vi "Main.vi"(8 "Error in":errorcluster) -> (0 "error out":errorcluster)   [LabVIEW 2018, in "Module B.lvlib"]
uses:
  Module B.lvlib
  Private/ctl/Message Data--cluster.ctl
  Private/ctl/State--enum.ctl
  Common/Common.lvlib
panel:
  out "Msg":string
  in  "Shut module A":bool
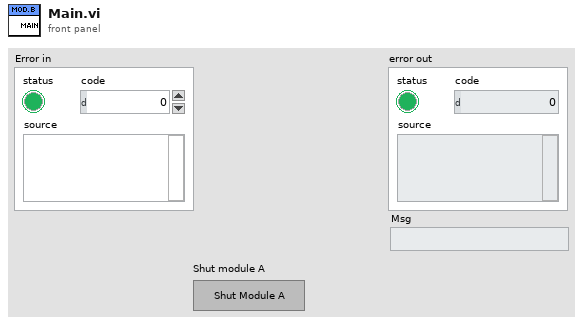
[diagram p1: front panel]
types:
  T1 = typedef "Module B.lvlib/Message Data--cluster.ctl" = cluster{"State":T2, "Data":variant}
  T2 = typedef "Module B.lvlib/State--enum.ctl" = enum16{"Initialize", "Error", "Shut Down", "Stop Module", "---", "Template", "Shut Module A"}
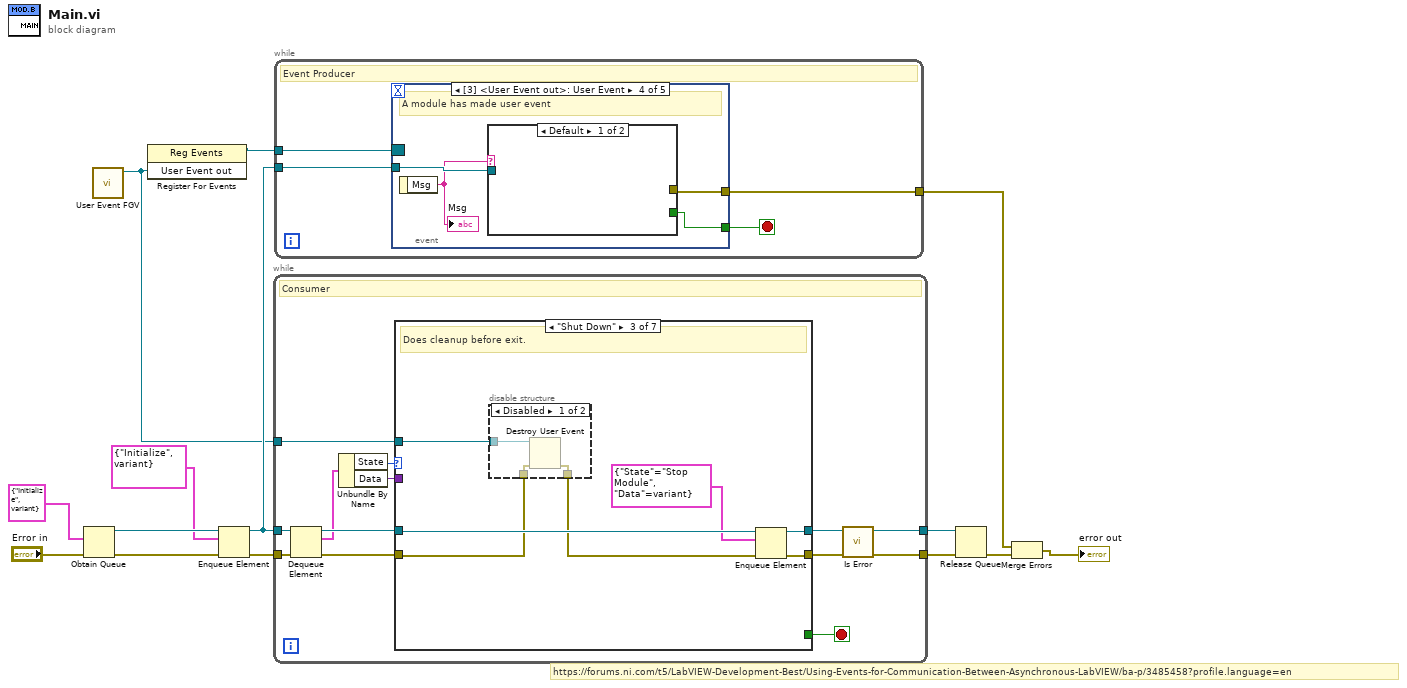
[diagram p0: block diagram]
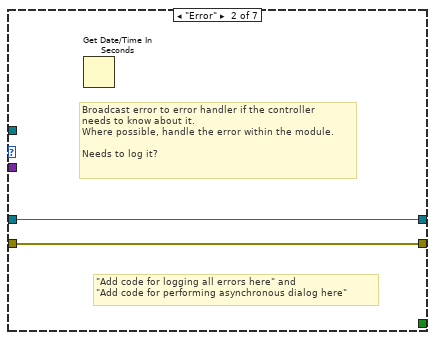
[diagram p3: hidden frame]
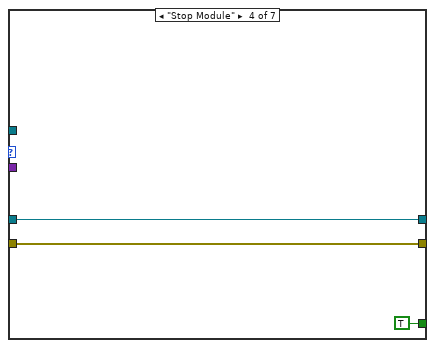
[diagram p5: hidden frame]
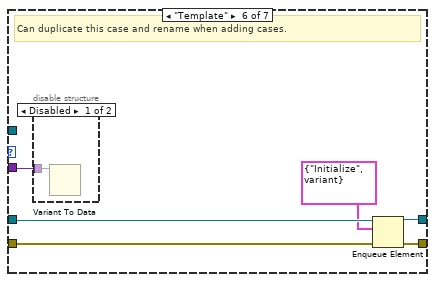
[diagram p7: hidden frame]
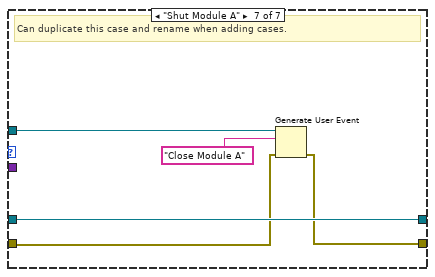
[diagram p9: hidden frame]
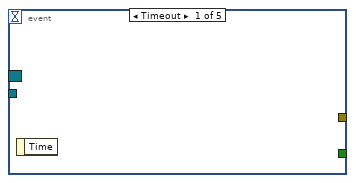
[diagram p10: hidden frame]
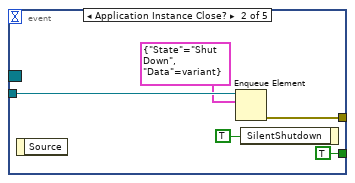
[diagram p11: hidden frame]
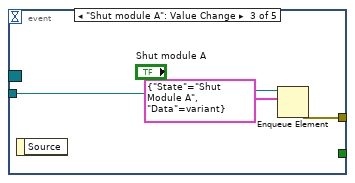
[diagram p12: hidden frame]
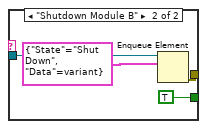
[diagram p13: hidden frame]
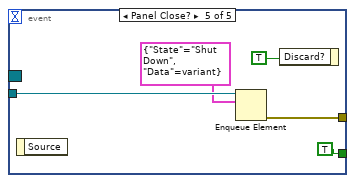
[diagram p14: hidden frame]
diagram:
  # "https://forums.ni.com/t5/LabVIEW-Development-Best/Using-Events-for-Communication-Between-Asynchronous-LabVIEW/ba-p/3485458?profile.language=en"
  n1 = Obtain Queue(element data type=T1 {"State"=enum."Initialize", "Data"=variant} ("Message Data--cluster"), error in (no error)="Error in") -> (queue out=w9:refnum<queue>, error out=w14:errorcluster)  [unwired: 3 in, 1 out]
  n2 = call "User Event FGV.vi"() -> ("User Event out"=w1:refnum<user-event>)  [unwired: 11 in]
  n3 = register-events(w1) -> (reference out=w2:refnum<event-registration>)  [unwired: 2 in, 1 out]
  n4 = Enqueue Element(queue=w9, element=T1 {"State"=enum."Initialize", "Data"=variant}, error in (no error)=w14) -> (queue out=w8:refnum<queue>, error out=w13:errorcluster)  [unwired: 1 in, 1 out]
  n5 = while {
    tunnel: w8 -> [w27]
    tunnel: w13 -> [w26]
    tunnel: [w18] -> w11
    tunnel: [w19] -> w10
    tunnel: w1 -> [w15]
    stop <- w16 stop-if-true
    # "Consumer"
    n6 = Dequeue Element(queue=w27, error in (no error)=w26) -> (queue out=w25:refnum<queue>, element=w24:T1, error out=w22:errorcluster)  [unwired: 1 in, 1 out]
    n7 = Unbundle By Name(w24) -> ("State"=w23:T2, "Data"=w21:variant)
    n8 = case shown="\"Shut Down\"" w23 {
      tunnel: w25 -> [w29 w31 w38 w44 w47 w50 w59]
      tunnel: [w29 w31 w37 w44 w47 w51 w59] -> w17
      tunnel: w22 -> [w28 w30 w33 w43 w46 w49 w57]
      tunnel: [w28 w30 w36 w43 w46 w52 w58] -> w20
      tunnel: w21 -> [_ _ _ _ _ w53 _]
      tunnel: [_ _ _ TRUE _ _ _] -> w16
      tunnel: w15 -> [_ _ w34 _ _ _ w56]
      frame "Initialize", Default {
      }
      frame "Error" {
        # "\"Add code for logging all errors here\" and \n\"Add code for performing asynchronous dialog here\""
        # "Broadcast error to error handler if the controller \nneeds to know about it.\nWhere possible, handle the error within the module.\n\nNeeds to log it?"
        n9 = Get Date/Time In Seconds() -> ()  [unwired: 1 out]
      }
      frame "Shut Down" {
        # "Does cleanup before exit."
        n10 = disable-structure shown="Disabled" {
          disable-tunnel: w34 -> [w41 _]
          disable-tunnel: w33 -> [w40 w42]
          disable-tunnel: [w39 w42] -> w32
          frame Disabled {
            n11 = Destroy User Event(user event=w41, error in=w40) -> (error out=w39:errorcluster)
          }
          frame Enabled {
          }
        }
        n12 = Enqueue Element(queue=w38, element=T1 {"State"=enum."Stop Module", "Data"=variant}, error in (no error)=w32) -> (queue out=w37:refnum<queue>, error out=w36:errorcluster)  [unwired: 1 in, 1 out]
      }
      frame "Stop Module" {
      }
      frame "---" {
        # "Divider - no code."
      }
      frame "Template" {
        # "Can duplicate this case and rename when adding cases."
        n13 = disable-structure shown="Disabled" {
          disable-tunnel: w53 -> [w54 _]
          frame Disabled {
            n14 = Variant To Data(Variant=w54) -> ()  [unwired: 2 in, 2 out]
          }
          frame Enabled {
          }
        }
        n15 = Enqueue Element(queue=w50, element=T1 {"State"=enum."Initialize", "Data"=variant}, error in (no error)=w49) -> (queue out=w51:refnum<queue>, error out=w52:errorcluster)  [unwired: 1 in, 1 out]
      }
      frame "Shut Module A" {
        # "Can duplicate this case and rename when adding cases."
        n16 = Generate User Event(user event=w56, event data cluster="Close Module A" ("event data"), error in=w57) -> (error out=w58:errorcluster)  [unwired: 1 in, 1 out]
      }
    }
    n17 = call "Is Error.vi"("error in"=w20, "Queue in"=w17) -> ("error out"=w19:errorcluster, "Queue out"=w18:refnum<queue>)  [unwired: 8 in]
  }
  n18 = while {
    tunnel: w8 -> [w63]
    tunnel: [w62] -> w3
    tunnel: w2 -> [w60]
    stop <- w61 stop-if-true
    # "Event Producer"
    n19 = event shown="[3] <User Event out>: User Event" {
      selector: w60 -> [_ _ _ _ _]
      dyn-events: _ -> [_ _ _ _ _]
      timeout: _ -> [_ _ _ _ _]
      tunnel: w63 -> [_ w66 w71 w74 w82]
      tunnel: [_ w67 w70 w75 w83] -> w62
      tunnel: [_ TRUE _ w72 TRUE] -> w61
      event Timeout {
        n20 = event-data() -> ()  [unwired: 1 in, 1 out]
      }
      event Application Instance Close? {
        n21 = event-data() -> ()  [unwired: 1 in, 1 out]
        n22 = Enqueue Element(queue=w66, element=T1 {"State"=enum."Shut Down", "Data"=variant}) -> (error out=w67:errorcluster)  [unwired: 2 in, 2 out]
        n23 = event-data("SilentShutdown"=TRUE) -> ()  [unwired: 1 in, 1 out]
      }
      event "Shut module A": Value Change {
        n24 = event-data() -> ()  [unwired: 1 in, 1 out]
        n25 = Enqueue Element(queue=w71, element=T1 {"State"=enum."Shut Module A", "Data"=variant}) -> (error out=w70:errorcluster)  [unwired: 2 in, 2 out]
      }
      event User Event {
        # "A module has made user event"
        n26 = event-data() -> ("Msg"=w73:string)  [unwired: 1 in]
        "Msg" <- w73
        n27 = case shown="Default" w73 {
          tunnel: [_ w79] -> w75
          tunnel: w74 -> [_ w78]
          tunnel: [_ TRUE] -> w72
          frame Default {
          }
          frame "Shutdown Module B" {
            n28 = Enqueue Element(queue=w78, element=T1 {"State"=enum."Shut Down", "Data"=variant}) -> (error out=w79:errorcluster)  [unwired: 2 in, 2 out]
          }
        }
      }
      event Panel Close? {
        n29 = event-data() -> ()  [unwired: 1 in, 1 out]
        n30 = Enqueue Element(queue=w82, element=T1 {"State"=enum."Shut Down", "Data"=variant}) -> (error out=w83:errorcluster)  [unwired: 2 in, 2 out]
        n31 = event-data("Discard?"=TRUE ("SilentShutdown")) -> ()  [unwired: 1 in, 1 out]
      }
    }
  }
  n32 = Release Queue(queue=w11, error in (no error)=w10) -> (error out=w4:errorcluster)  [unwired: 1 in, 2 out]
  n33 = Merge Errors(w3, w4) -> (→"error out":errorcluster)
